vi "Useful Values.vi"() -> ()   [LabVIEW 2013]
panel:
  in  "Arm Setpoint":dbl
  in  "Arm Offset":dbl
  in  "Intake Setpoint":dbl
  in  "About to Shoot":bool
  in  "Teleop Time":dbl=2.48
  in  "Comp?":bool
  in  "Just Shot":bool
  in  "Arm Cal?":bool
  in  "Right Motors":dbl
  in  "Left Motors":dbl
  in  "Angluar Rate":dbl
  in  "Angle":dbl
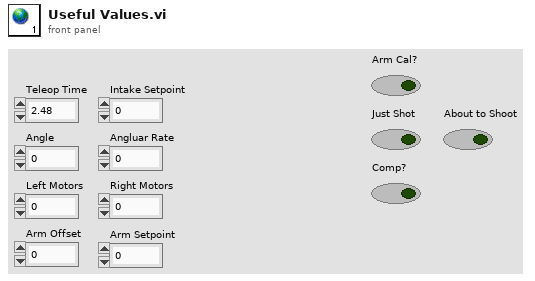
[diagram p1: front panel]
diagram:
